vi "DtCreateDOutChan.vi"(5 "Board Name":string, 9 "Port Number":u32, 11 "error in (no error)":errorcluster) -> (4 "Task out":i32, 15 "error out":errorcluster)   [LabVIEW 2022 SP3]
doc: "Creates one or more virtual digital output ports that you can update."
uses:
  DtLvLink.lvlib
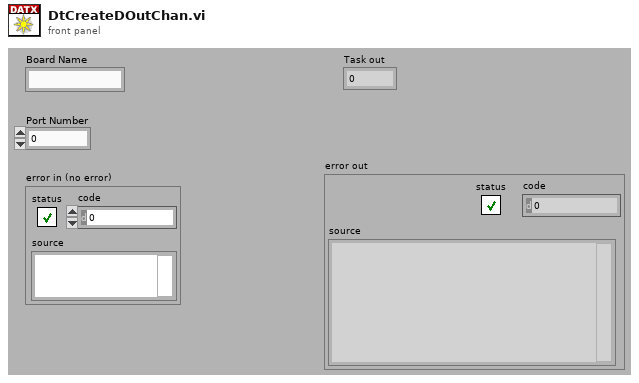
[diagram p1: front panel]
types:
  T1 = enum32{"AnalogInput", "AnalogOutput", "DigitalInput", "DigitalOutput", "Quadrature", "CounterTimer"}
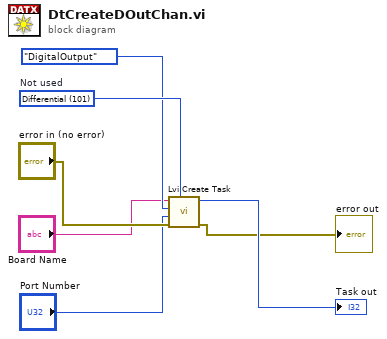
[diagram p0: block diagram]
diagram:
  w7 = 101 items=["SingleEnded"=100, "Differential"=101]  # Not used
  n1 = call "Lvi Create Task.vi"("SEorDiff"=w7, "error in (no error)"="error in (no error)", "SubSysIndex"="Port Number", "ChanType"=T1."DigitalOutput", "BoardName"="Board Name") -> ("error out"=→"error out":errorcluster, "TaskRef"=→"Task out":i32)  [unwired: 4 in, 1 out]
